vi "INI hexaxes and wait until finished.vi"(0 "System no.":i32=1 min=1 max=4 step=1, 2 "INI hexapod?":bool, 3 "INI sep. axes":string[](array[string]), 4 "Timeout, sec":u32=90, 5 "error in":errorcluster, 12 "Stop refnum":refnum<vi>) -> (14 "Hexapod initialized?":bool, 15 "Sep. axes initialized?":bool[](array[boolean]), 16 "Stopped?":bool, 19 "error out":errorcluster)   [LabVIEW 2020]
doc: "Initializes hexapod and/or additional axes and waits until procedure has finished, Stop refnum or Local stop is TRUE or a timeout condition has occured. When using as a sub-VI, use Stop refnum to stop VI from caller.\n\nC-887, F-206, M-8X0: Only for GCS syntax version = GCS 1.0 (Check with CSV?.vi. If CSV?.vi is not supported, syntax version is GCS 1.0).\nGCS 1.0: Since version 4.0.0 of the F-206 firmware and version 4.5.0 of the M-8X0 firmware it is possible to stop the ini procedure by sending #24. \nGCS 2.0 or higher: VI calls FRF instead for compatibility."
uses:
  General command.llb/Global2 (Array).vi
  General command.llb/Controller names.ctl
  Communication.llb/Global1.vi
  Communication.llb/Syntax.ctl
panel:
  in  "Local stop":bool
  # "Initializes hexapod and/or additional axes and waits until \nprocedure has finished, Stop refnum or Local stop is TRUE\nor a timeout condition has occured."
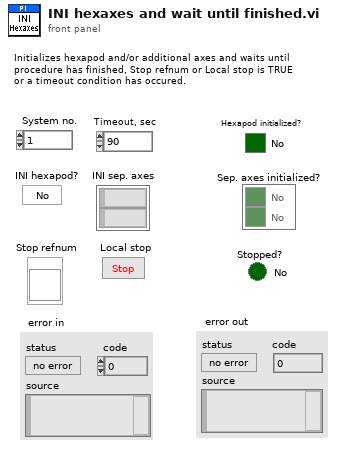
[diagram p1: front panel]
types:
  T1 = typedef "Syntax.ctl" = enum16{"GCS 1.0", "GCS 2.0", "GCS 3.0"}
  T2 = typedef "Controller names.ctl" = enum16{"None", "Analog", "C-702", "C-413", "C-414", "C-843", "C-843.PM", "C-844", "C-848", "C-865", "C-866", "C-867", "C-877", "C-880", "C-884", "C-885", "C-886", "C-887", "C-891", "E-135", "E-516", "E-517", "E-518", "E-709", "E-710", "E-712", "E-725", "E-727", "E-753", "E-754", "E-755", "E-761", "E-816", "E-861", "E-870", "E-871", "E-872", "E-873", "E-874", "F-206", "HydraPollux", "M-840", "M-850", "M-8X0", "Mercury", "Mercury_GCS", "PI_GCS2"}
  T3 = cluster{"Conn. axes":string[], "Controller name":T2}[]
  T4 = cluster{"Conn. axes":string[], "Controller name":T2}
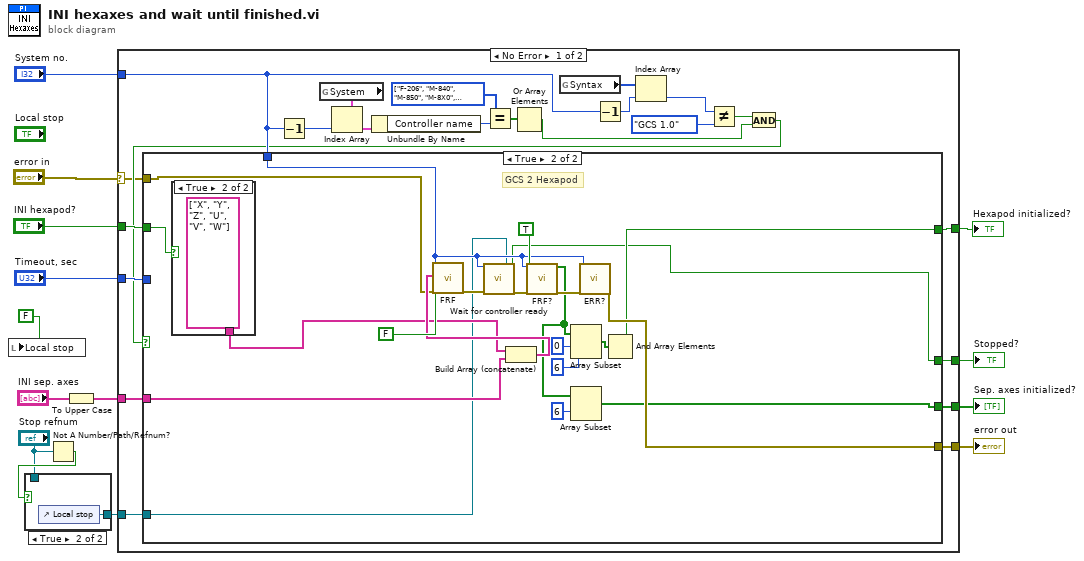
[diagram p0: block diagram]
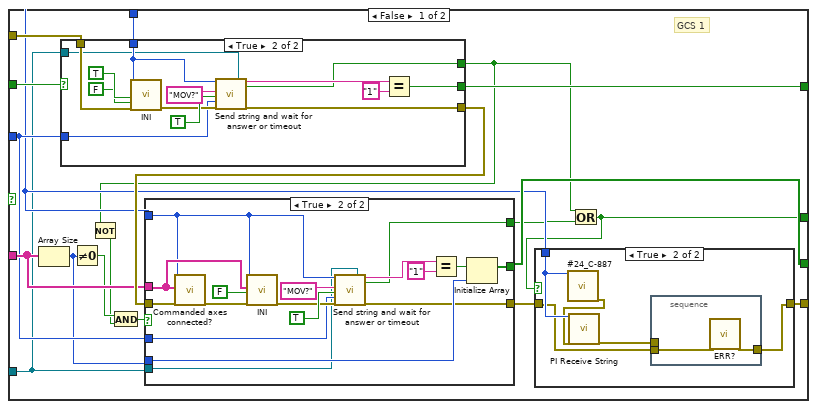
[diagram p3: hidden frame]
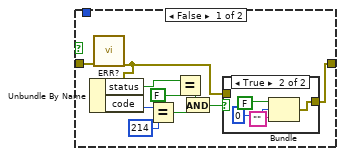
[diagram p4: hidden frame]
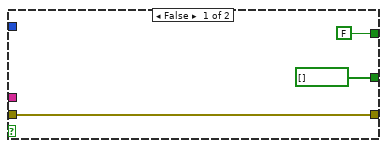
[diagram p6: hidden frame]
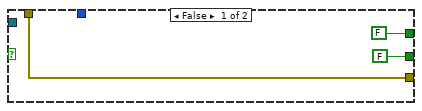
[diagram p7: hidden frame]
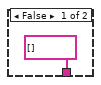
[diagram p8: hidden frame]
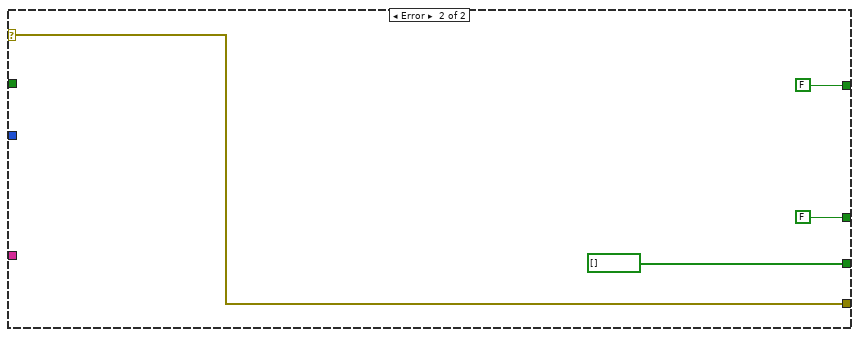
[diagram p9: hidden frame]
diagram:
  n1 = local write "Local stop"(FALSE ("Local stop")) -> ()
  n2 = Not A Number/Path/Refnum?(number/path/refnum="Stop refnum") -> (NaN/Path/Refnum?=w6:bool)
  n3 = case shown="True" w6 {
    tunnel: "Stop refnum" -> [w15 _]
    tunnel: [w15 w16] -> w3
    frame False {
    }
    frame True {
      n4 = control-ref of="Local stop"() -> (w16:refnum<vi>)
    }
  }
  n5 = To Upper Case(1:"INI sep. axes") -> (0:w9:string[])
  n6 = case shown="No Error" "error in" {
    selector: "error in" -> [w18 w140]
    tunnel: "System no." -> [w22 _]
    tunnel: "INI hexapod?" -> [w37 _]
    tunnel: [w34 w140] -> w12
    tunnel: "Timeout, sec" -> [w38 _]
    tunnel: w9 -> [w39 _]
    tunnel: [w36 FALSE] -> w8
    tunnel: [w35 bool[] []] -> w7
    tunnel: w3 -> [w33 _]
    tunnel: [w32 FALSE] -> w2
    frame No Error {
      w30 = T2[] [enum."F-206", enum."M-840", enum."M-850", enum."M-8X0", enum."C-887"] items=["None", "Analog", "C-702", "C-413", "C-414", "C-843", "C-843.PM", "C-844", "C-848", "C-865", "C-866", "C-867", "C-877", "C-880", "C-884", "C-885", "C-886", "C-887", "C-891", "E-135", "E-516", "E-517", "E-518", "E-709", "E-710", "E-712", "E-725", "E-727", "E-753", "E-754", "E-755", "E-761", "E-816", "E-861", "E-870", "E-871", "E-872", "E-873", "E-874", "F-206", "HydraPollux", "M-840", "M-850", "M-8X0", "Mercury", "Mercury_GCS", "PI_GCS2"]
      n7 = Decrement(x=w22) -> (x-1=w19:i32)
      n8 = global read "Global2 (Array).vi" "System"() -> (w27:T3)
      n9 = Index Array(array=w27, index=w19) -> (element=w28:T4)
      n10 = Unbundle By Name(w28) -> ("Controller name"=w29:T2)
      n11 = Equal?(x=w30, y=w29) -> (x = y?=w31:bool[])
      n12 = Or Array Elements(Boolean array=w31) -> (logical OR=w21:bool)
      n13 = global read "Global1.vi" "Syntax"() -> (w26:T1[])
      n14 = Decrement(x=w22) -> (x-1=w25:i32)
      n15 = Index Array(array=w26, index=w25) -> (element=w24:T1)
      n16 = Not Equal?(x=w24, y=Syntax."GCS 1.0") -> (x != y?=w23:bool)
      n17 = And(x=w23, y=w21) -> (x .and. y?=w20:bool)
      n18 = case shown="True" w20 {
        tunnel: w18 -> [w57 w128]
        tunnel: w39 -> [w55 w127]
        tunnel: w38 -> [w54 _]
        tunnel: w37 -> [w52 w123]
        tunnel: [w51 w122] -> w36
        tunnel: [w50 w118] -> w35
        tunnel: w22 -> [w49 w125]
        tunnel: [w47 w129] -> w34
        tunnel: w33 -> [w46 w124]
        tunnel: [w40 w117] -> w32
        frame False {
          # "GCS 1"
          n19 = Array Size(array=w55) -> (size(s)=w53:i32)
          n20 = case shown="True" w52 {
            tunnel: w49 -> [_ w113]
            tunnel: w57 -> [w102 w114]
            tunnel: w54 -> [_ w109]
            tunnel: [w102 w107] -> w56
            tunnel: [FALSE w106] -> w51
            tunnel: w46 -> [_ w103]
            tunnel: [FALSE ("Stopped?") w105] -> w43
            frame False {
            }
            frame True {
              n21 = call "INI.vi"("Connection"=w113, 3:TRUE ("All axes?"), 4:FALSE ("Axis identifier?"), "error in"=w114) -> ("error out"=w110:errorcluster)  [unwired: 15 out]
              n22 = call "Send string and wait for answer or timeout.vi"("System no."=w113, "String to send"="MOV?", "Attach Linefeed?"=TRUE, "Timeout, sec"=w109, "error in"=w110, "Stop refnum"=w103) -> ("String read"=w108:string, "Stopped?"=w105:bool, "error out"=w107:errorcluster)  [unwired: 3 in, 8 out]
              n23 = Equal?(x=w108, y="1") -> (x = y?=w106:bool)
            }
          }
          n24 = Not Equal To 0?(x=w53) -> (x != 0?=w44:bool)
          n25 = Not(x=w43) -> (.not. x?=w42:bool)
          n26 = And(x=w44, y=w42) -> (x .and. y?=w41:bool)
          n27 = case shown="True" w41 {
            tunnel: w56 -> [w82 w99]
            tunnel: w55 -> [_ w98]
            tunnel: w49 -> [_ w92]
            tunnel: w54 -> [_ w91]
            tunnel: w53 -> [_ w89]
            tunnel: [w82 w88] -> w48
            tunnel: [bool[] [] w87] -> w50
            tunnel: w46 -> [_ w85]
            tunnel: [FALSE ("Stopped?") w84] -> w45
            frame False {
            }
            frame True {
              n28 = call "Commanded axes connected?.vi"("System no."=w92, "Commanded axes"=w98, "error in"=w99) -> ("error out"=w97:errorcluster)  [unwired: 1 in, 15 out]
              n29 = call "INI.vi"("Connection"=w92, 2:w98, 3:FALSE ("All axes?"), "error in"=w97) -> ("error out"=w93:errorcluster)  [unwired: 15 out]
              n30 = call "Send string and wait for answer or timeout.vi"("System no."=w92, "String to send"="MOV?", "Attach Linefeed?"=TRUE, "Timeout, sec"=w91, "error in"=w93, "Stop refnum"=w85) -> ("String read"=w94:string, "Stopped?"=w84:bool, "error out"=w88:errorcluster)  [unwired: 3 in, 8 out]
              n31 = Equal?(x=w94, y="1") -> (x = y?=w90:bool)
              n32 = Initialize Array(w90, w89) -> (w87:bool[])
            }
          }
          n33 = Or(x=w43, y=w45) -> (x .or. y?=w40:bool)
          n34 = case shown="True" w40 {
            tunnel: w49 -> [_ w77]
            tunnel: w48 -> [w67 w75]
            tunnel: [w58 w74] -> w47
            frame False {
              n35 = call "ERR?.vi"("error in"=w67) -> ("error out"=w59:errorcluster)  [unwired: 1 in, 17 out]
              n36 = Unbundle By Name(w59) -> ("status"=w66:bool, "code"=w64:i32)
              n37 = Equal?(x=w64, y=214) -> (x = y?=w62:bool)
              n38 = Equal?(x=w66, y=FALSE) -> (x = y?=w61:bool)
              n39 = And(x=w61, y=w62) -> (x .and. y?=w60:bool)
              n40 = case shown="True" w60 {
                tunnel: w59 -> [w68 _]
                tunnel: [w68 w69] -> w58
                frame False {
                }
                frame True {
                  n41 = Bundle(FALSE, 0, "") -> (w69:errorcluster)  [unwired: 1 out]
                }
              }
            }
            frame True {
              n42 = call "#24_C-887.vi"("System no."=w77) -> ("error out"=w76:errorcluster)  [unwired: 1 in, 17 out]
              n43 = call "PI Receive String.vi"("System no."=w77, "error in"=w76) -> ("error out"=w73:errorcluster)  [unwired: 1 in, 16 out]
              n44 = stacked-sequence {
                tunnel: w75 -> [w79]
                tunnel: [w78] -> w74
                tunnel: w73 -> [_]
                frame #0 {
                  n45 = call "ERR?.vi"("error in"=w79) -> ("error out"=w78:errorcluster)  [unwired: 1 in, 17 out]
                }
              }
            }
          }
        }
        frame True {
          # "GCS 2 Hexapod"
          n46 = case shown="True" w123 {
            tunnel: [string[] [] ("Conn. axes") string[] ["X", "Y", "Z", "U", "V", "W"] ("Conn. axes")] -> w126
            frame False {
            }
            frame True {
            }
          }
          n47 = Build Array (concatenate)(w126, w127) -> (w133:string[])
          n48 = call "FRF.vi"("System no."=w125, "Affected axes"=w133, "All axes?"=FALSE, "error in"=w128) -> ("error out"=w137:errorcluster)  [unwired: 1 in, 14 out]
          n49 = call "Wait for controller ready.vi"("System no."=w125, "error in"=w137, "Stop refnum"=w124) -> ("Stopped"=w117:bool, "error out"=w136:errorcluster)  [unwired: 1 in, 14 out]
          n50 = call "FRF?.vi"("System no."=w125, "All axes?"=TRUE, "error in"=w136) -> ("Referenced?"=w119:bool[], "error out"=w135:errorcluster)  [unwired: 2 in, 13 out]
          n51 = Array Subset(array=w119, index=0, length=6) -> (w130:bool[])
          n52 = Array Subset(array=w119, index=6 ("length")) -> (w118:bool[])  [unwired: 1 in]
          n53 = call "ERR?.vi"("System no."=w125, "error in"=w135) -> ("error out"=w129:errorcluster)  [unwired: 17 out]
          n54 = And Array Elements(Boolean array=w130) -> (logical AND=w122:bool)
        }
      }
    }
    frame Error {
    }
  }
  "error out" <- w12
  "Hexapod initialized?" <- w8
  "Sep. axes initialized?" <- w7
  "Stopped?" <- w2
